vi "Handle Timeout.vi"(8 "error in (no error)":errorcluster, 11 "cRIO Vacuum in":refnum<class "cRIO Vacuum.lvclass">) -> (0 "error out":errorcluster, 3 "cRIO Vacuum out":refnum<class "cRIO Vacuum.lvclass">)   [LabVIEW 2015, in "cRIO-Carbondioxide.lvlib" / "CO2-Actor.lvlib" / "cRIO Vacuum.lvclass"]
uses:
  cRIO Vacuum.lvclass
  cRIO Vacuum.lvclass/cRIO Vacuum.ctl
  Controls/Vacuum State Enumerator.ctl
  <vilib>/ptbypt/Time Domain.llb/Derivative x(t) PtByPt.vi
  <vilib>/ptbypt/NI_PtbyPt.lvlib
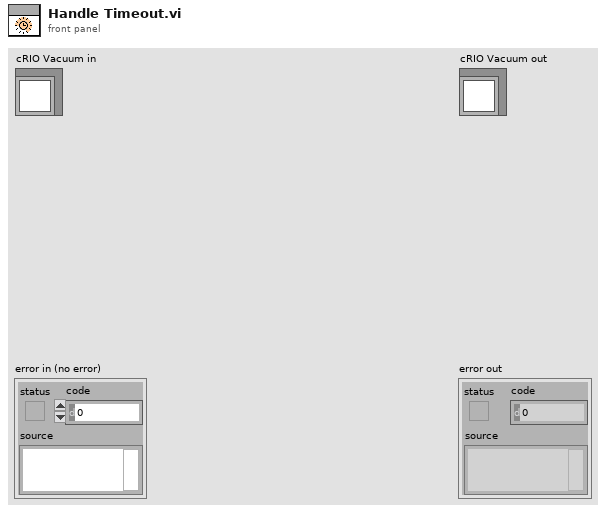
[diagram p1: front panel]
types:
  T1 = typedef "Vacuum State Enumerator.ctl" = enum16{"Pressure Rising", "Plateau", "Pressure Dropping", "Valley", "Low Valley", "Leak", "Unknown"}
  T2 = cluster{"Rizing":dbl, "Plateau":dbl, "Dropping":dbl, "Valley":dbl}
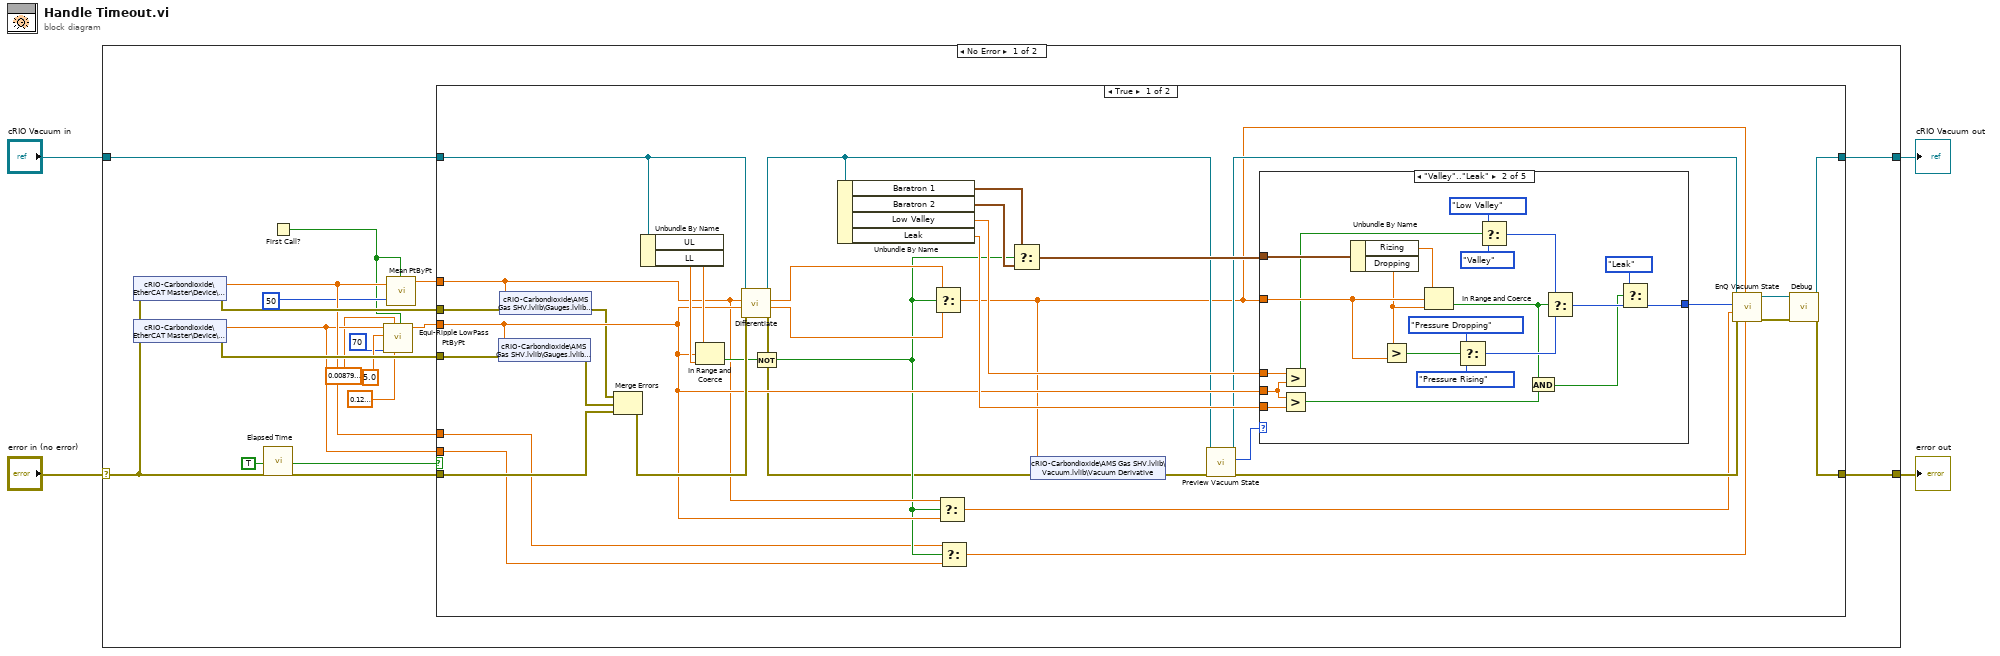
[diagram p0: block diagram]
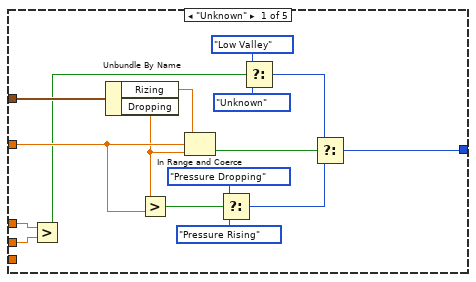
[diagram p2: hidden frame]
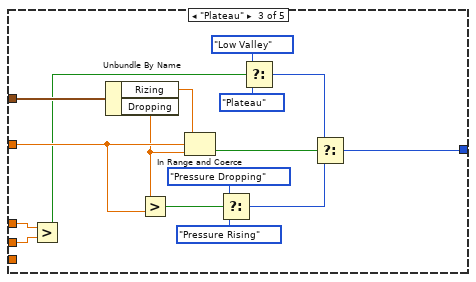
[diagram p3: hidden frame]
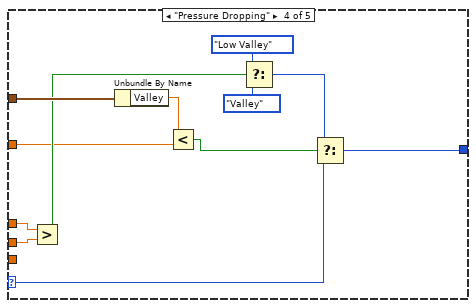
[diagram p4: hidden frame]
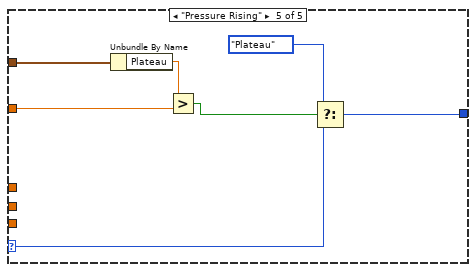
[diagram p5: hidden frame]
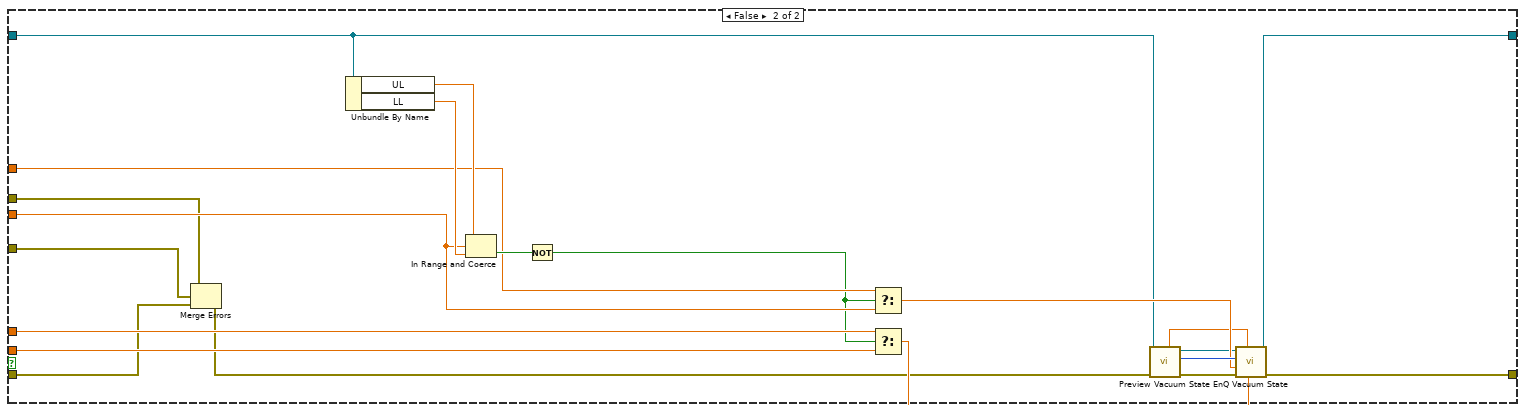
[diagram p6: hidden frame]
diagram:
  n1 = case shown="No Error" "error in (no error)" {
    selector: "error in (no error)" -> [w13 w154]
    tunnel: [w15 w154] -> w3
    tunnel: [w16 w153] -> w1
    tunnel: "cRIO Vacuum in" -> [w17 w153]
    frame No Error {
      n2 = shared-variable "cRIO-Carbondioxide\\EtherCAT Master\\Device\\Mod7\\Baratron 1"(error in=w13) -> (w14:dbl, error out=w21:errorcluster)
      n3 = shared-variable "cRIO-Carbondioxide\\EtherCAT Master\\Device\\Mod7\\Baratron 2"(error in=w13) -> (w11:dbl, error out=w22:errorcluster)
      n4 = call "Elapsed Time"("Auto Reset"=TRUE, "error in (no error)"=w13) -> ("Time has Elapsed"=w19:bool, "error out"=w23:errorcluster)  [unwired: 10 in, 6 out]
      n5 = First Call?() -> (First Call?: T/F=w9:bool)
      n6 = call <vilib>:"Equi-Ripple LowPass PtByPt.vi"("initialize"=w9, "stop freq"=0.1299999999999999, "pass freq"=0.00879999999999983, "# of taps"=70, "sampling freq: fs"=5.0, "x"=w11) -> ("Filtered x"=w10:dbl)  [unwired: 3 in, 1 out]
      n7 = call <vilib>:"Mean PtByPt.vi"("x"=w14, "sample length"=50, "initialize"=w9) -> ("mean"=w20:dbl)  [unwired: 1 in, 1 out]
      n8 = case shown="True" w19 {
        tunnel: w23 -> [w59 w137]
        tunnel: w22 -> [w58 w132]
        tunnel: w21 -> [w57 w133]
        tunnel: w20 -> [w42 w139]
        tunnel: w10 -> [w43 w138]
        tunnel: [w28 w140] -> w15
        tunnel: w17 -> [w27 w136]
        tunnel: [w30 w141] -> w16
        tunnel: w14 -> [w36 w146]
        tunnel: w11 -> [w35 w145]
        frame True {
          n9 = shared-variable "cRIO-Carbondioxide\\AMS Gas SHV.lvlib\\Gauges.lvlib\\Baratron 2"(w43, error in=w58) -> (error out=w56:errorcluster)
          n10 = shared-variable "cRIO-Carbondioxide\\AMS Gas SHV.lvlib\\Gauges.lvlib\\Baratron 1"(w42, error in=w57) -> (error out=w32:errorcluster)
          n11 = Merge Errors(w32, w56, w59) -> (w53:errorcluster)
          n12 = Unbundle By Name(w27) -> ("UL"=w55:dbl, "LL"=w54:dbl)
          n13 = In Range and Coerce(upper limit=w55, x=w43, lower limit=w54) -> (In Range?=w47:bool)  [unwired: 1 out]
          n14 = call "Differentiate.vi"("error in (no error)"=w53, "Baratron 2"=w43, "Baratron 1"=w42, "cRIO Vacuum in"=w27) -> ("error out"=w26:errorcluster, "d/dt 2"=w51:dbl, "d/dt 1"=w52:dbl, "cRIO Vacuum out"=w33:refnum<class "cRIO Vacuum.lvclass">)  [unwired: 4 in]
          n15 = Not(x=w47) -> (.not. x?=w37:bool)
          n16 = Unbundle By Name(w33) -> ("Baratron 1"=w50:T2, "Baratron 2"=w49:T2, "Low Valley"=w45:dbl, "Leak"=w44:dbl)
          n17 = Select(t=w52, s=w37, f=w51) -> (s? t:f=w24:dbl)
          n18 = Select(t=w42, s=w37, f=w43) -> (s? t:f=w38:dbl)
          n19 = Select(t=w36, s=w37, f=w35) -> (s? t:f=w34:dbl)
          n20 = Select(t=w50, s=w37, f=w49) -> (s? t:f=w48:T2)
          n21 = shared-variable "cRIO-Carbondioxide\\AMS Gas SHV.lvlib\\Vacuum.lvlib\\Vacuum Derivative"(w24, error in=w26) -> (error out=w25:errorcluster)
          n22 = call "Preview Vacuum State.vi"("error in (no error)"=w25, "cRIO Vacuum in"=w33) -> ("error out"=w41:errorcluster, "Vacuum State"=w46:T1, "cRIO Vacuum out"=w39:refnum<class "cRIO Vacuum.lvclass">)  [unwired: 3 in, 4 out]
          n23 = case shown="\"Valley\"..\"Leak\"" w46 {
            selector: w46 -> [_ _ _ w113 w126]
            tunnel: w48 -> [w75 w96 w112 w124 w131]
            tunnel: w24 -> [w71 w93 w108 w115 w128]
            tunnel: w43 -> [w65 w84 w102 w122 _]
            tunnel: w45 -> [w66 w88 w103 w123 _]
            tunnel: [w60 w79 w97 w117 w130] -> w40
            tunnel: w44 -> [_ w83 _ _ _]
            frame "Unknown" {
              n24 = Greater?(x=w66, y=w65) -> (0:w64:bool)
              n25 = Unbundle By Name(w75) -> ("Rizing"=w74:dbl, "Dropping"=w70:dbl)
              n26 = Greater?(x=w70, y=w71) -> (0:w72:bool)
              n27 = In Range and Coerce(upper limit=w74, x=w71, lower limit=w70) -> (In Range?=w73:bool)  [unwired: 1 out]
              n28 = Select(t=Vacuum_State_Enumerator."Pressure Dropping" ("Vacuum State"), s=w72, f=Vacuum_State_Enumerator."Pressure Rising") -> (s? t:f=w69:T1)
              n29 = Select(t=Vacuum_State_Enumerator."Low Valley", s=w64, f=Vacuum_State_Enumerator."Unknown" ("Vacuum State")) -> (s? t:f=w61:T1)
              n30 = Select(t=w61, s=w73, f=w69) -> (s? t:f=w60:T1)
            }
            frame "Valley".."Leak" {
              n31 = Greater?(x=w88, y=w84) -> (0:w87:bool)
              n32 = Greater?(x=w84, y=w83) -> (0:w78:bool)
              n33 = Unbundle By Name(w96) -> ("Rizing"=w95:dbl, "Dropping"=w92:dbl)
              n34 = Greater?(x=w92, y=w93) -> (0:w94:bool)
              n35 = In Range and Coerce(upper limit=w95, x=w93, lower limit=w92) -> (In Range?=w77:bool)  [unwired: 1 out]
              n36 = Select(t=Vacuum_State_Enumerator."Pressure Dropping" ("Vacuum State"), s=w94, f=Vacuum_State_Enumerator."Pressure Rising") -> (s? t:f=w91:T1)
              n37 = Select(t=Vacuum_State_Enumerator."Low Valley", s=w87, f=Vacuum_State_Enumerator."Valley" ("Vacuum State")) -> (s? t:f=w81:T1)
              n38 = And(x=w77, y=w78) -> (x .and. y?=w76:bool)
              n39 = Select(t=w81, s=w77, f=w91) -> (s? t:f=w80:T1)
              n40 = Select(t=Vacuum_State_Enumerator."Leak", s=w76, f=w80) -> (s? t:f=w79:T1)
            }
            frame "Plateau" {
              n41 = Greater?(x=w103, y=w102) -> (0:w101:bool)
              n42 = Unbundle By Name(w112) -> ("Rizing"=w111:dbl, "Dropping"=w107:dbl)
              n43 = Greater?(x=w107, y=w108) -> (0:w109:bool)
              n44 = In Range and Coerce(upper limit=w111, x=w108, lower limit=w107) -> (In Range?=w110:bool)  [unwired: 1 out]
              n45 = Select(t=Vacuum_State_Enumerator."Pressure Dropping" ("Vacuum State"), s=w109, f=Vacuum_State_Enumerator."Pressure Rising") -> (s? t:f=w106:T1)
              n46 = Select(t=Vacuum_State_Enumerator."Low Valley", s=w101, f=Vacuum_State_Enumerator."Plateau" ("Vacuum State")) -> (s? t:f=w98:T1)
              n47 = Select(t=w98, s=w110, f=w106) -> (s? t:f=w97:T1)
            }
            frame "Pressure Dropping" {
              n48 = Greater?(x=w123, y=w122) -> (0:w121:bool)
              n49 = Unbundle By Name(w124) -> ("Valley"=w116:dbl)
              n50 = Less?(x=w116, y=w115) -> (x < y?=w114:bool)
              n51 = Select(t=Vacuum_State_Enumerator."Low Valley", s=w121, f=Vacuum_State_Enumerator."Valley" ("Vacuum State")) -> (s? t:f=w118:T1)
              n52 = Select(t=w118, s=w114, f=w113) -> (s? t:f=w117:T1)
            }
            frame "Pressure Rising" {
              n53 = Unbundle By Name(w131) -> ("Plateau"=w129:dbl)
              n54 = Greater?(x=w129, y=w128) -> (0:w127:bool)
              n55 = Select(t=Vacuum_State_Enumerator."Plateau", s=w127, f=w126) -> (s? t:f=w130:T1)
            }
          }
          n56 = call "EnQ Vacuum State.vi"("Raw Pressure"=w34, "d/dt"=w24, "error in (no error)"=w41, "Pressure"=w38, "State"=w40, "cRIO Vacuum in"=w39) -> ("error out"=w29:errorcluster, "cRIO Vacuum out"=w31:refnum<class "cRIO Vacuum.lvclass">)  [unwired: 4 out]
          n57 = call "Debug.vi"("error in (no error)"=w29, "cRIO Vacuum in"=w31) -> ("error out"=w28:errorcluster, "cRIO Vacuum out"=w30:refnum<class "cRIO Vacuum.lvclass">)  [unwired: 8 in]
        }
        frame False {
          n58 = Merge Errors(w133, w132, w137) -> (w134:errorcluster)
          n59 = Unbundle By Name(w136) -> ("UL"=w152:dbl, "LL"=w151:dbl)
          n60 = In Range and Coerce(upper limit=w152, x=w138, lower limit=w151) -> (In Range?=w150:bool)  [unwired: 1 out]
          n61 = Not(x=w150) -> (.not. x?=w135:bool)
          n62 = Select(t=w139, s=w135, f=w138) -> (s? t:f=w147:dbl)
          n63 = Select(t=w146, s=w135, f=w145) -> (s? t:f=w144:dbl)
          n64 = call "Preview Vacuum State.vi"("error in (no error)"=w134, "cRIO Vacuum in"=w136) -> ("error out"=w149:errorcluster, "Vacuum State"=w148:T1, "cRIO Vacuum out"=w142:refnum<class "cRIO Vacuum.lvclass">, "d/dt"=w143:dbl)  [unwired: 3 in, 3 out]
          n65 = call "EnQ Vacuum State.vi"("Raw Pressure"=w144, "d/dt"=w143, "error in (no error)"=w149, "Pressure"=w147, "State"=w148, "cRIO Vacuum in"=w142) -> ("error out"=w140:errorcluster, "cRIO Vacuum out"=w141:refnum<class "cRIO Vacuum.lvclass">)  [unwired: 4 out]
        }
      }
    }
    frame Error {
    }
  }
  "error out" <- w3
  "cRIO Vacuum out" <- w1
